vi "Logic.vi"(9 "x":bool, 13 "y":bool) -> (10 "x .and. y":bool)   [LabVIEW 2015]
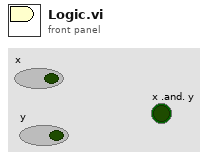
[diagram p1: front panel]
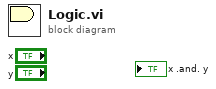
[diagram p0: block diagram]
diagram:
